vi "NumOfPhases.vi"(8 "Error In":errorcluster, 11 "Phases":T1(array[cluster]) {"Phase Select" items=["Phase ALL", "Phase A", "Phase B", "Phase C"]}) -> (0 "Error Out":errorcluster, 3 "NumberOfPhases>3":bool)   [LabVIEW 2018, in "AcPwrPlugins.lvlib" / "ChromaAcLoad.lvclass"]
uses:
  ChromaAcLoad.lvclass
  <vilib>/Utility/error.llb/Error Cluster From Error Code.vi
  <vilib>/ErrorRing/Error Ring.xnode
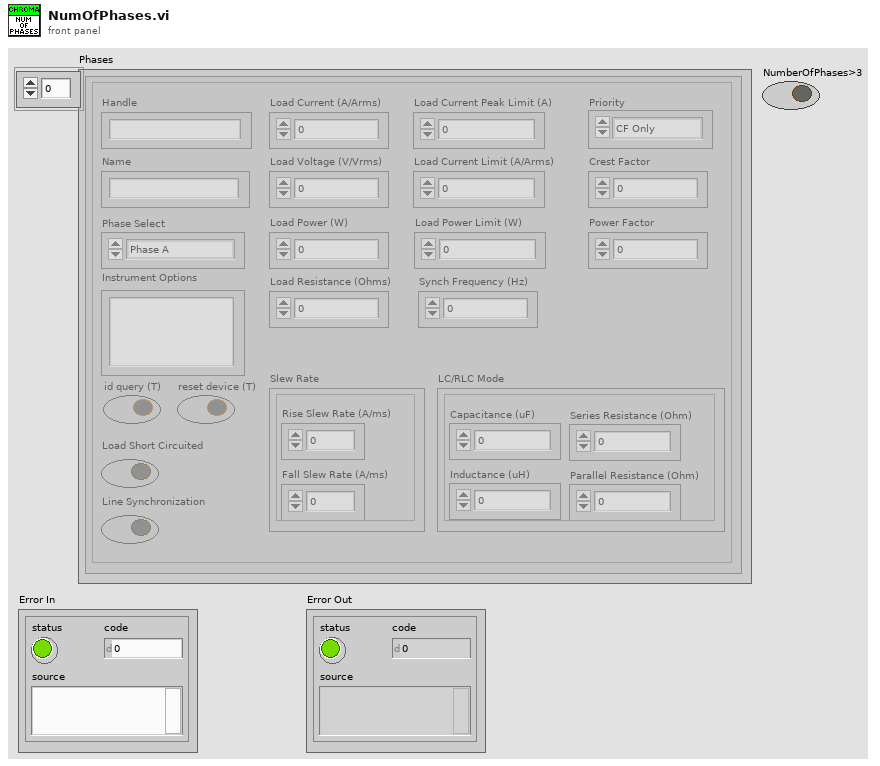
[diagram p1: front panel]
types:
  T1 = cluster{"Handle":string, "Name":string, "Phase Select":i32, "Instrument Options":string, "id query (T)":bool, "reset device (T)":bool, "Load Short Circuited":bool, "Line Synchronization":bool, "Load Current (A/Arms)":dbl, "Load Voltage (V/Vrms)":dbl, "Load Power (W)":dbl, "Load Resistance (Ohms)":dbl, "Load Current Peak Limit (A)":dbl, "Load Current Limit (A/Arms)":dbl, "Load Power Limit (W)":dbl, "Synch Frequency (Hz)":dbl, "Priority":enum16{"CF Only", "PF Only", "Both (CF)", "Both (PF)"}, "Crest Factor":dbl, "Power Factor":dbl, "Slew Rate":cluster{"Rise Slew Rate (A/ms)":i32, "Fall Slew Rate (A/ms)":i32}, "LC/RLC Mode":cluster{"Capacitance (uF)":i32, "Inductance (uH)":i32, "Series Resistance (Ohm)":dbl, "Parallel Resistance (Ohm)":dbl}, "Timing":cluster{"TimingOn":enum16{""}, "Hours":u32, "Minutes":u32, "Seconds":dbl, "CutoffVoltage":dbl}, "Connected":bool}[]
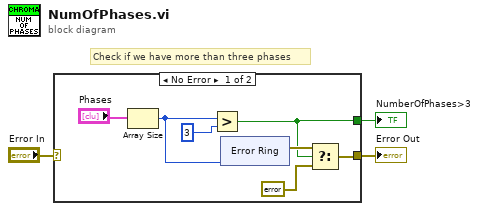
[diagram p0: block diagram]
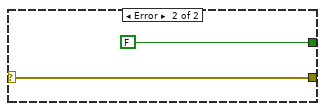
[diagram p2: hidden frame]
diagram:
  # "Check if we have more than three phases"
  n1 = case shown="No Error" "Error In" {
    selector: "Error In" -> [_ w19]
    tunnel: [w6 w19] -> w2
    tunnel: [w5 FALSE] -> w1
    frame No Error {
      n2 = Array Size(array="Phases") -> (size(s)=w9:i32)
      n3 = Greater?(x=w9, y=3) -> (0:w5:bool)
      n4 = xnode "Error Ring"("parameter 0"=w9) -> ("error out"=w8:errorcluster)
      n5 = Select(t=w8, s=w5, f=errorcluster {"status"=FALSE, "code"=0, "source"=""}) -> (s? t:f=w6:errorcluster)
    }
    frame Error {
    }
  }
  "Error Out" <- w2
  "NumberOfPhases>3" <- w1
